vi "Kinesis-program-one-motor.vi"() -> ()   [LabVIEW 2014]
doc: "André Romero - 2017\nandretec@ifsc.usp.br"
panel:
  out "GetPOS":dbl format="%#_6e"
  out "Numeric":i32
  out "IsMoving":bool
  out "GetPOS X":dbl=10.0 format="%^#1_6e"
  in  "GO Move":bool
  out "Motor 1":bool
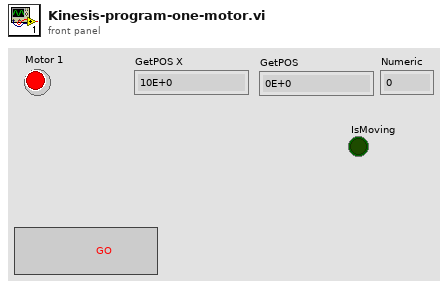
[diagram p1: front panel]
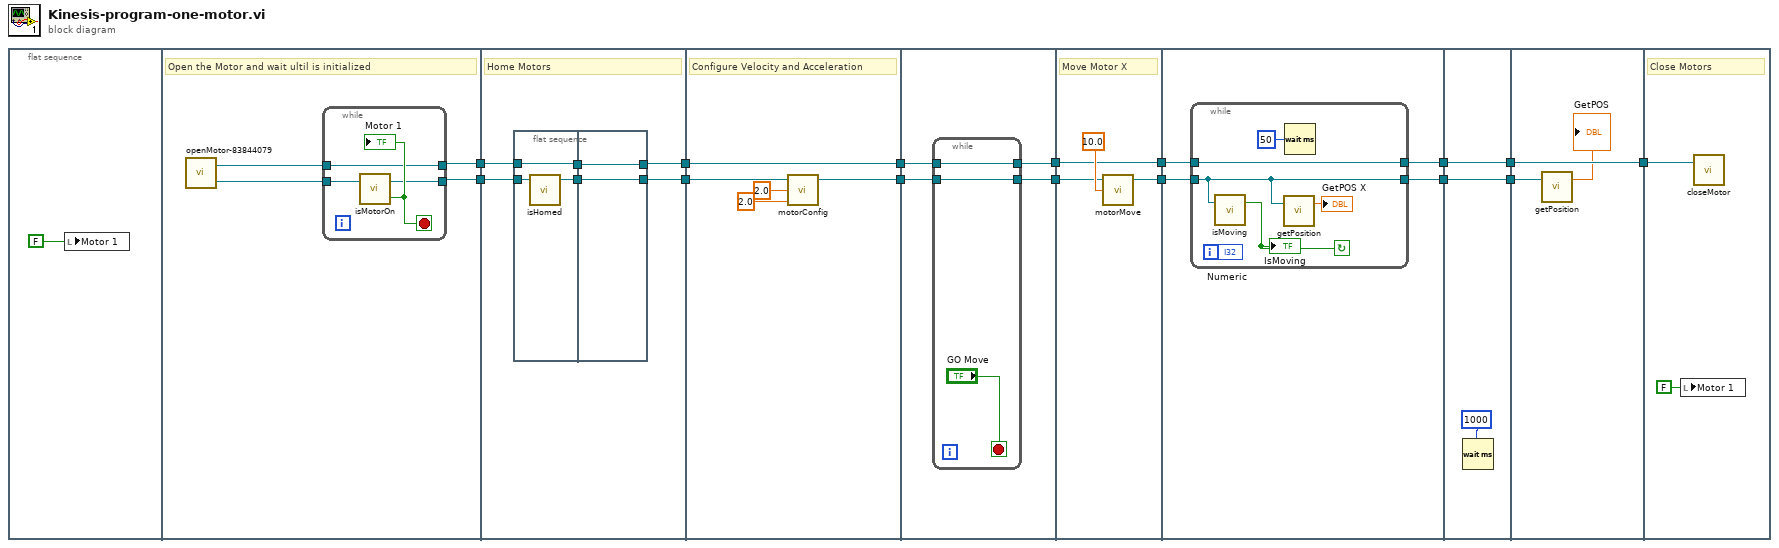
[diagram p0: block diagram]
diagram:
  n1 = flat-sequence {
    tunnel: [w20] -> w2
    tunnel: [w19] -> w1
    tunnel: w2 -> [w30]
    tunnel: w1 -> [w29]
    tunnel: [w27] -> w15
    tunnel: [w26] -> w13
    tunnel: w15 -> [w40]
    tunnel: [w40] -> w14
    tunnel: w13 -> [w36]
    tunnel: [w37] -> w12
    tunnel: w14 -> [w44]
    tunnel: [w43] -> w10
    tunnel: w12 -> [w41]
    tunnel: [w42] -> w11
    tunnel: w11 -> [w49]
    tunnel: [w48] -> w9
    tunnel: w10 -> [w50]
    tunnel: [w50] -> w8
    tunnel: w9 -> [w52]
    tunnel: [w53] -> w7
    tunnel: w8 -> [w55]
    tunnel: [w54] -> w6
    tunnel: w7 -> [w64]
    tunnel: [w64] -> w5
    tunnel: w6 -> [w63]
    tunnel: [w63] -> w4
    tunnel: w5 -> [w66]
    tunnel: w4 -> [w67]
    tunnel: [w67] -> w3
    tunnel: w3 -> [w69]
    frame #0 {
      n2 = local write "Motor 1"(FALSE ("isConnected")) -> ()
    }
    frame #1 {
      # "Open the Motor and wait ultil is initialized"
      n3 = call "openMotor-83844079.vi"() -> ("Device"=w18:refnum<k24>, ".NET Refnum out"=w17:refnum<k24>)  [unwired: 2 in]
      n4 = while {
        tunnel: [w23] -> w20
        tunnel: [w21] -> w19
        tunnel: w17 -> [w23]
        tunnel: w18 -> [w22]
        stop <- w24 stop-if-true
        n5 = call "isMotorOn.vi"("Device"=w22) -> ("isConnected"=w24:bool, "Device out"=w21:refnum<k24>)  [unwired: 1 in]
        "Motor 1" <- w24
      }
    }
    frame #2 {
      # "Home Motors"
      n6 = flat-sequence {
        tunnel: w30 -> [w33]
        tunnel: w29 -> [w32]
        tunnel: [w33] -> w28
        tunnel: [w31] -> w25
        tunnel: [w34] -> w26
        tunnel: [w35] -> w27
        tunnel: w28 -> [w35]
        tunnel: w25 -> [w34]
        frame #0 {
          n7 = call "isHomed.vi"("Device in"=w32) -> ("Device out"=w31:refnum<k24>)  [unwired: 4 in]
        }
        frame #1 {
        }
      }
    }
    frame #3 {
      # "Configure Velocity and Acceleration"
      n8 = call "motorConfig.vi"("Velocity"=2.0 ("MaxVelocity"), "Acceleration"=2.0, "Device in"=w36) -> ("Device out"=w37:refnum<k24>)  [unwired: 2 in]
    }
    frame #4 {
      n9 = while {
        tunnel: [w46] -> w43
        tunnel: w44 -> [w46]
        tunnel: [w45] -> w42
        tunnel: w41 -> [w45]
        stop <- "GO Move" stop-if-true
      }
    }
    frame #5 {
      # "Move Motor X"
      n10 = call "motorMove.vi"("position"=10.0, "Device in"=w49) -> ("Device out"=w48:refnum<k24>)  [unwired: 3 in]
    }
    frame #6 {
      n11 = while {
        tunnel: w55 -> [w61]
        tunnel: w52 -> [w60]
        tunnel: [w61] -> w54
        tunnel: [w60] -> w53
        i -> [w57]
        stop <- w59 continue-if-true
        n12 = call "isMoving.vi"("Device in"=w60) -> ("IsMoving"=w59:bool)  [unwired: 2 in]
        "IsMoving" <- w59
        n13 = call "getPosition.vi"("Device"=w60) -> ("GetPOS"=→"GetPOS X":dbl)  [unwired: 2 in]
        n14 = Wait (ms)(milliseconds to wait=u32 50) -> ()  [unwired: 1 out]
        "Numeric" <- w57
      }
    }
    frame #7 {
      n15 = Wait (ms)(milliseconds to wait=u32 1000) -> ()  [unwired: 1 out]
    }
    frame #8 {
      n16 = call "getPosition.vi"("Device"=w66) -> ("GetPOS"=→"GetPOS":dbl)  [unwired: 2 in]
    }
    frame #9 {
      # "Close Motors"
      n17 = local write "Motor 1"(FALSE ("Motor 1")) -> ()
      n18 = call "closeMotor.vi"(".NET Refnum in"=w69) -> ()  [unwired: 2 in]
    }
  }
